vi "setCamRamAllocation.vi"(0 "Camera in":refnum<class "Camera.lvclass">, 5 "percents":u32[](array[numeric]), 11 "error in (no error)":errorcluster) -> (4 "Camera out":refnum<class "Camera.lvclass">, 15 "error out":errorcluster)   [LabVIEW 2019, in "Camera.lvclass"]
doc: "For cameras with internal memory (CAMRAM) this VI can be used to set the number of images allocated to each of the four segments. Allocation is specified as a percentage of the total, so the sum of the allocation elements cannot exceed 100. The total can be less than 100, i.e. not all memory is allocated."
uses:
  Camera.lvclass
  Camera.lvclass/Camera.ctl
  pco.sdk/StorageControl/StorageControl.lvlib
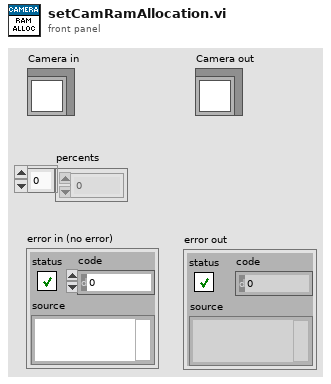
[diagram p1: front panel]
types:
  T1 = cluster{"dwRamSize":u32, "wPageSize":u16, "dwRamSegSize":u32[], "wActSeg":u16}
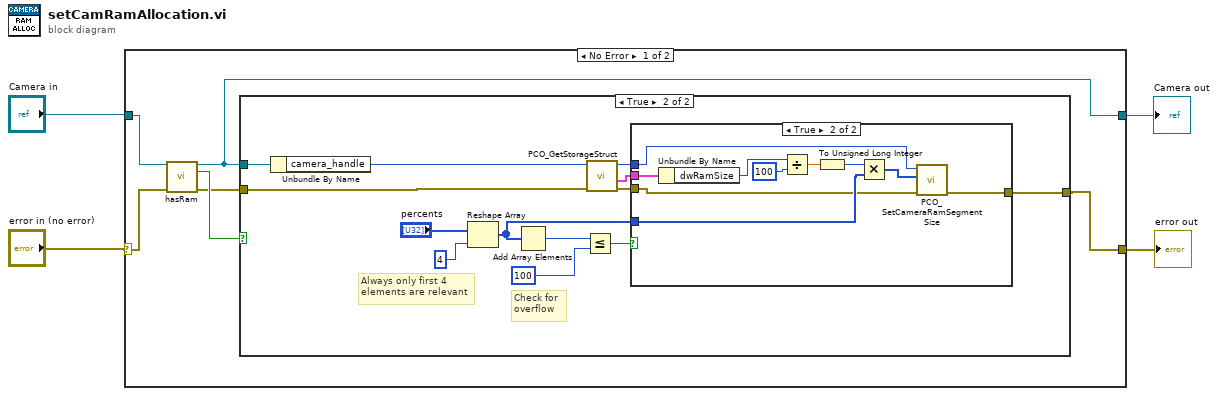
[diagram p0: block diagram]
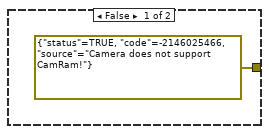
[diagram p2: hidden frame]
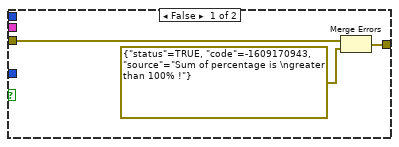
[diagram p3: hidden frame]
diagram:
  n1 = case shown="No Error" "error in (no error)" {
    selector: "error in (no error)" -> [w9 w39]
    tunnel: [w5 w39] -> w2
    tunnel: [w6 w38] -> w3
    tunnel: "Camera in" -> [w10 w38]
    frame No Error {
      n2 = call-dynamic "hasRam.vi"("Camera in"=w10, "error in (no error)"=w9) -> ("Camera out"=w6:refnum<class "Camera.lvclass">, "hasRam"=w8:bool, "error out"=w7:errorcluster)  [unwired: 11 in]
      n3 = case shown="True" w8 {
        tunnel: w6 -> [_ w24]
        tunnel: [errorcluster {"status"=TRUE, "code"=-2146025466, "source"="Camera does not support CamRam!"} ("error constant") w12] -> w5
        tunnel: w7 -> [_ w22]
        frame False {
        }
        frame True {
          # "Check for\noverflow"
          # "Always only first 4 \nelements are relevant"
          n4 = Unbundle By Name(w24) -> ("camera_handle"=w23:u64)
          n5 = Reshape Array("percents", 4 ("index")) -> (w16:u32[])
          n6 = Add Array Elements(numeric array=w16) -> (sum=w19:u32)
          n7 = Less Or Equal?(x=w19, y=u32 100) -> (x <= y?=w17:bool)
          n8 = call "PCO_GetStorageStruct.vi"("error in (no error)"=w22, "ph"=w23) -> ("error out"=w15:errorcluster, "strStorage"=w13:T1, "ph out"=w14:u64)  [unwired: 6 in, 1 out]
          n9 = case shown="True" w17 {
            tunnel: w16 -> [_ w33]
            tunnel: w15 -> [w26 w29]
            tunnel: w14 -> [_ w31]
            tunnel: w13 -> [_ w34]
            tunnel: [w25 w28] -> w12
            frame False {
              n10 = Merge Errors(w26, errorcluster {"status"=TRUE, "code"=-1609170943, "source"="Sum of percentage is \ngreater than 100% !"} ("error constant")) -> (w25:errorcluster)
            }
            frame True {
              n11 = Unbundle By Name(w34) -> ("dwRamSize"=w37:u32)
              n12 = Divide(x=w37, y=u32 100) -> (x/y=w35:dbl)
              n13 = To Unsigned Long Integer(number=w35) -> (unsigned 32bit integer=w32:u32)
              n14 = Multiply(x=w32, y=w33) -> (x*y=w30:u32[])
              n15 = call "PCO_SetCameraRamSegmentSize.vi"("error in (no error)"=w29, "dwRamSegSize"=w30, "ph"=w31) -> ("error out"=w28:errorcluster)  [unwired: 6 in, 2 out]
            }
          }
        }
      }
    }
    frame Error {
    }
  }
  "error out" <- w2
  "Camera out" <- w3
